vi "RemoveQandP.vi"(0 "Subtract Ped?":bool=TRUE, 4 "Qcurve":dbl[](array[numeric]), 5 "Raw data":dbl[](array[numeric])) -> (1 "Ped L-R":dbl, 2 "Corrected data":dbl[](array[numeric]), 3 "Ped Offfset":dbl format="%#_13g")   [LabVIEW 2018]
uses:
  Global 2.vi
panel:
  # "Subtracts Q curve and pedestal fron raw data"
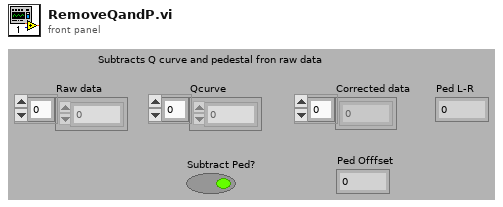
[diagram p1: front panel]
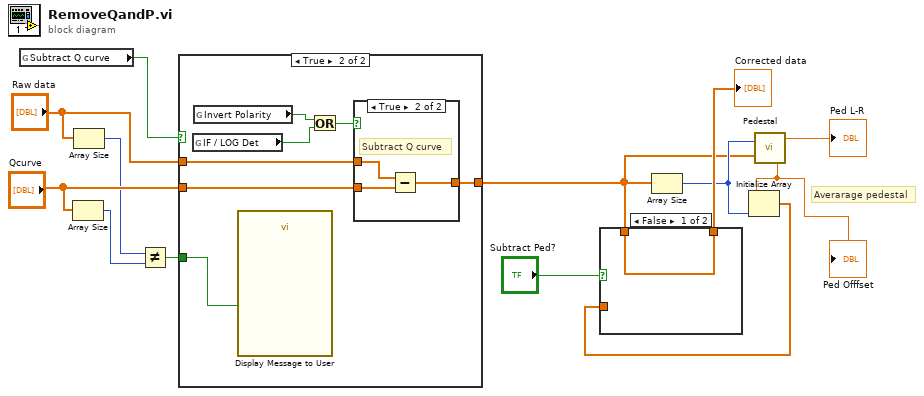
[diagram p0: block diagram]
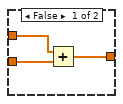
[diagram p3: hidden frame]
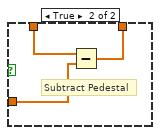
[diagram p4: hidden frame]
diagram:
  # "Averarage pedestal"
  n1 = global read "Global 2.vi" "Subtract Q curve"() -> (w2:bool)
  n2 = Array Size(array="Qcurve") -> (size(s)=w5:i32)
  n3 = Array Size(array="Raw data") -> (size(s)=w6:i32)
  n4 = Not Equal?(x=w6, y=w5) -> (x != y?=w1:bool)
  n5 = case shown="True" w2 {
    tunnel: [w14 w21] -> w10
    tunnel: "Raw data" -> [w14 w17]
    tunnel: "Qcurve" -> [_ w16]
    tunnel: w1 -> [_ w15]
    frame False {
    }
    frame True {
      n6 = global read "Global 2.vi" "IF / LOG Det"() -> (w19:bool)
      n7 = global read "Global 2.vi" "Invert Polarity"() -> (w20:bool)
      n8 = call "Display Message to User"("Enable"=w15) -> ()  [unwired: 9 in, 2 out]
      n9 = Or(x=w20, y=w19) -> (x .or. y?=w18:bool)
      n10 = case shown="True" w18 {
        tunnel: w17 -> [w23 w27]
        tunnel: [w22 w26] -> w21
        tunnel: w16 -> [w24 w25]
        frame False {
          n11 = Add(x=w23, y=w24) -> (x+y=w22:dbl[])
        }
        frame True {
          # "Subtract Q curve"
          n12 = Subtract(x=w27, y=w25) -> (x-y=w26:dbl[])
        }
      }
    }
  }
  n13 = Array Size(array=w10) -> (size(s)=w11:i32)
  n14 = call "Pedestal.vi"("Varray"=w10, "ArraySize"=w11) -> ("Average"=w4:dbl, "L-R"=→"Ped L-R":dbl)
  "Ped Offfset" <- w4
  n15 = Initialize Array(w4, w11) -> (w12:dbl[])
  n16 = case shown="False" "Subtract Ped?" {
    tunnel: [w28 w31] -> w13
    tunnel: w12 -> [_ w30]
    tunnel: w10 -> [w28 w29]
    frame False {
    }
    frame True {
      # "Subtract Pedestal"
      n17 = Subtract(x=w29, y=w30) -> (x-y=w31:dbl[])
    }
  }
  "Corrected data" <- w13
